vi "loadCoreCtls.vi"(10 "ControlsOnPage":refnum<vi>[](array[refnum]), 11 "Base path":path) -> (0 "error out":errorcluster, 3 "path out":path)   [LabVIEW 2016]
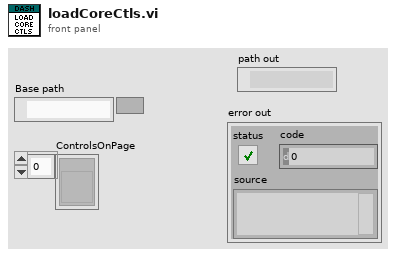
[diagram p1: front panel]
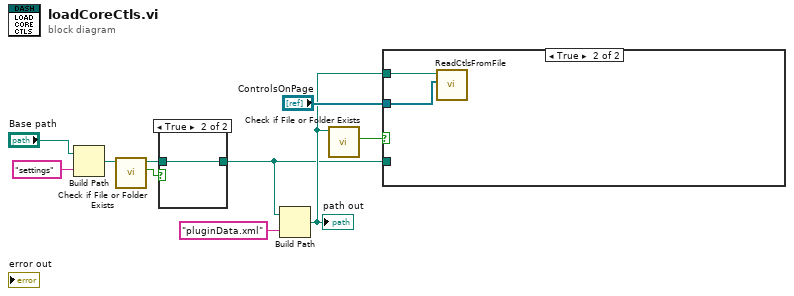
[diagram p0: block diagram]
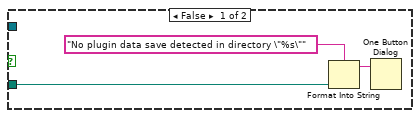
[diagram p2: hidden frame]
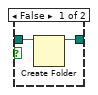
[diagram p3: hidden frame]
diagram:
  n1 = Build Path(base path="Base path", name or relative path="settings") -> (appended path=w3:path)
  n2 = call <vilib>:"Check if File or Folder Exists.vi"("path"=w3) -> ("file or folder exists?"=w4:bool, "dup path"=w5:path)  [unwired: 8 in, 1 out]
  n3 = case shown="True" w4 {
    tunnel: w5 -> [w12 w13]
    tunnel: [w11 w13] -> w7
    frame False {
      n4 = Create Folder(path (use dialog)=w12) -> (created path=w11:path)  [unwired: 2 in, 2 out]
    }
    frame True {
    }
  }
  n5 = Build Path(base path=w7, name or relative path="pluginData.xml") -> (appended path=w8:path)
  "path out" <- w8
  n6 = call <vilib>:"Check if File or Folder Exists.vi"("path"=w8) -> ("file or folder exists?"=w6:bool)  [unwired: 8 in, 2 out]
  n7 = case shown="True" w6 {
    tunnel: "ControlsOnPage" -> [_ w18]
    tunnel: w8 -> [_ w17]
    tunnel: w7 -> [w15 _]
    frame False {
      n8 = Format Into String(format string="No plugin data save detected in directory \"%s\"" ("message"), w15) -> (resulting string=w14:string)  [unwired: 2 in, 1 out]
      n9 = One Button Dialog(message=w14) -> ()  [unwired: 1 in, 1 out]
    }
    frame True {
      n10 = call "ReadCtlsFromFile.vi"("ControlsToLoad"=w18, "selected path"=w17) -> ()  [unwired: 9 in, 1 out]
    }
  }
